vi "unmarshalling.vi"(7 "Type":variant, 8 "error in (no error)":errorcluster, 10 "String":string, 11 "Serializer":refnum<class "Serializer.PlainText.INI.lvclass">) -> (0 "error out":errorcluster, 2 "Variant":variant, 3 "Serializer out":refnum<class "Serializer.PlainText.INI.lvclass">)   [LabVIEW 2013, in "OpenSerializer.lvlib" / "Serializer.PlainText.INI.lvclass"]
uses:
  Serializer.PlainText.INI.lvclass
  <vilib>/LabVIEW Open Source Project/Data Manipulation/TypeDescriptor/TypeDescriptor_GetName.vi
  <vilib>/LabVIEW Open Source Project/Data Manipulation/TypeDescriptor/TypeDescriptor_GetType.vi
  <vilib>/LabVIEW Open Source Project/Data Manipulation/TypeDescriptor/TypeDescriptor_GetPString.vi
  <vilib>/Utility/VariantDataType/VariantType.lvlib
  <vilib>/LabVIEW Open Source Project/Data Manipulation/Variant/OpenVariant.lvlib
  Serializer.PlainText/Serializer.PlainText.lvclass
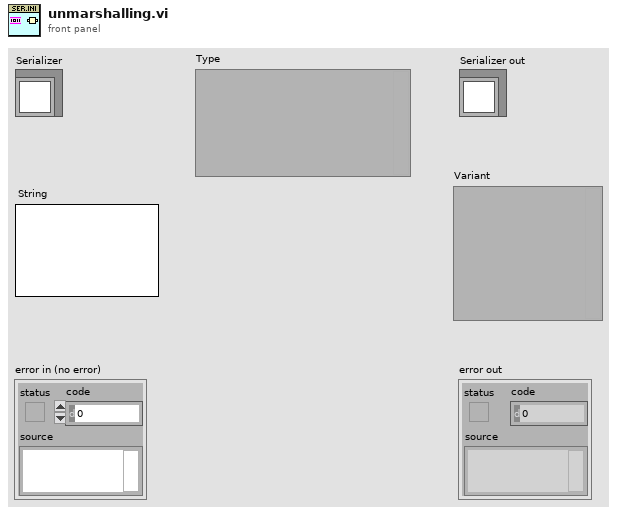
[diagram p1: front panel]
types:
  T1 = typedef "VariantType.lvlib/Type.ctl" = enum8{"Invalid Type", "Void", "I8", "I16", "I32", "I64", "U8", "U16", "U32", "U64", "Single Float", "Double Float", "Extended Float", "Single Complex", "Double Complex", "Extended Complex", "Enum U8", "Enum U16", "Enum U32", "Enum U64", "Single Float With Unit", "Double Float With Unit", "Extended Float With Unit", "Single Complex with Unit", "Double Complex with Unit", "Extended Complex with Unit", "Boolean", "String", "Path", "Picture", "Tag", "Array", "Cluster", "Variant", "LV Variant", "Waveform", "Timestamp", "Digital Waveform", "Digital Data", "ExpressData", "Refnum", "External Data", "VI", "Poly VI", "LabVIEW Class Instance", "Fixed Point"}
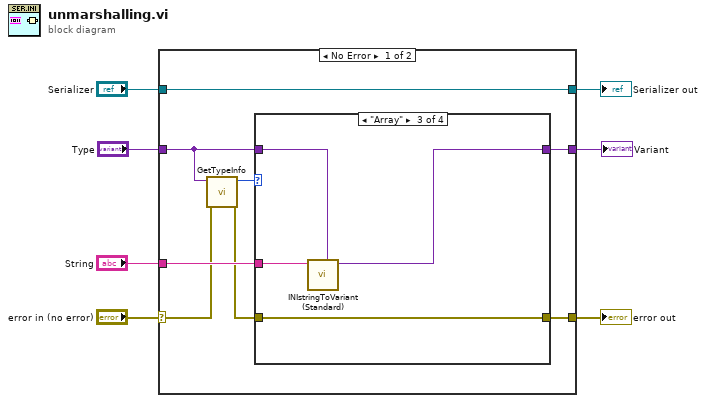
[diagram p0: block diagram]
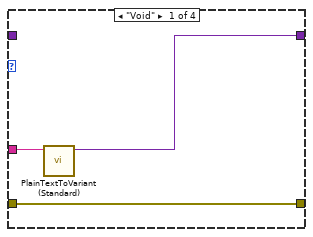
[diagram p2: hidden frame]
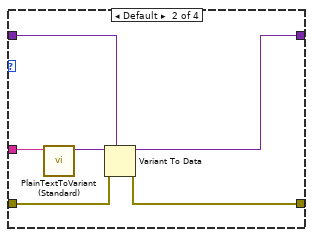
[diagram p3: hidden frame]
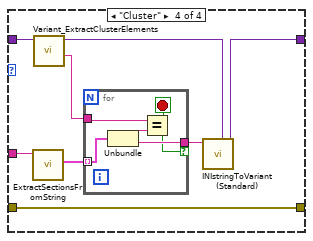
[diagram p4: hidden frame]
diagram:
  n1 = case shown="No Error" "error in (no error)" {
    selector: "error in (no error)" -> [w10 w43]
    tunnel: [w12 w43] -> w6
    tunnel: [w8 w42] -> w4
    tunnel: "Serializer" -> [w8 w42]
    tunnel: [w15 _] -> w3
    tunnel: "Type" -> [w14 _]
    tunnel: "String" -> [w11 _]
    frame No Error {
      n2 = call <vilib>:"GetTypeInfo.vi"("error in (no error)"=w10, "Variant"=w14) -> ("error out"=w9:errorcluster, "Type Enum"=w13:T1)  [unwired: 5 in, 3 out]
      n3 = case shown="\"Array\"" w13 {
        tunnel: [w16 w21 w25 w29] -> w15
        tunnel: w14 -> [_ w22 w26 w34]
        tunnel: w9 -> [w18 w20 w28 w33]
        tunnel: [w18 w19 w28 w33] -> w12
        tunnel: w11 -> [w17 w24 w27 w32]
        frame "Void" {
          n4 = call "PlainTextToVariant (Standard).vi"("String-formatted Value"=w17) -> ("Variant-formatted Value"=w16:variant)  [unwired: 9 in, 1 out]
        }
        frame Default {
          n5 = call "PlainTextToVariant (Standard).vi"("String-formatted Value"=w24) -> ("Variant-formatted Value"=w23:variant)  [unwired: 9 in, 1 out]
          n6 = Variant To Data(error in=w20, type=w22, Variant=w23) -> (data=w21:variant, error out=w19:errorcluster)
        }
        frame "Array" {
          n7 = call "INIstringToVariant (Standard).vi"("type"=w26, "INI Content"=w27) -> ("Variant-formatted Value"=w25:variant)  [unwired: 8 in, 1 out]
        }
        frame "Cluster" {
          n8 = call "ExtractSectionsFromString.vi"("String"=w32) -> ("Sections"=w36:cluster{"key":string, "value":string}[])  [unwired: 9 in, 1 out]
          n9 = call <vilib>:"Variant_ExtractClusterElements.vi"("Cluster"=w34) -> ("name"=w35:string, "Cluster dup"=w30:variant)  [unwired: 8 in, 1 out]
          n10 = for {
            tunnel: w36 -> [w41] mode=indexing
            tunnel: w35 -> [w40]
            tunnel: [w38] -> w31 if=w37
            stop <- w37 stop-if-true
            n11 = Unbundle(w41) -> ("key"=w39:string, "value"=w38:string)
            n12 = Equal?(x=w40, y=w39) -> (x = y?=w37:bool)
          }
          n13 = call "INIstringToVariant (Standard).vi"("type"=w30, "INI Content"=w31) -> ("Variant-formatted Value"=w29:variant)  [unwired: 8 in, 1 out]
        }
      }
    }
    frame Error {
    }
  }
  "error out" <- w6
  "Serializer out" <- w4
  "Variant" <- w3
